vi "ReadREPL.vi"(8 "error in (no error)":errorcluster, 11 "Python":T1) -> (0 "error out":errorcluster, 1 "bytes read":u32, 2 "String":string, 3 "Python":T1)   [LabVIEW 2022 SP3]
uses:
  PythonCtrl.ctl
  Processors.ctl
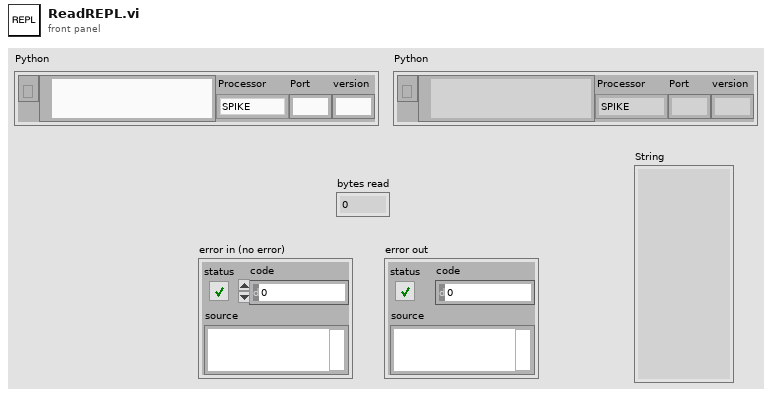
[diagram p1: front panel]
types:
  T1 = typedef "PythonCtrl.ctl" = cluster{"session":refnum<k35>, "PyPath":path, "Processor":T2, "Port":string, "version":string}
  T2 = typedef "Processors.ctl" = enum16{"SPIKE", "Pi", "Pi_ssh", "OpenMV", "Dunio"}
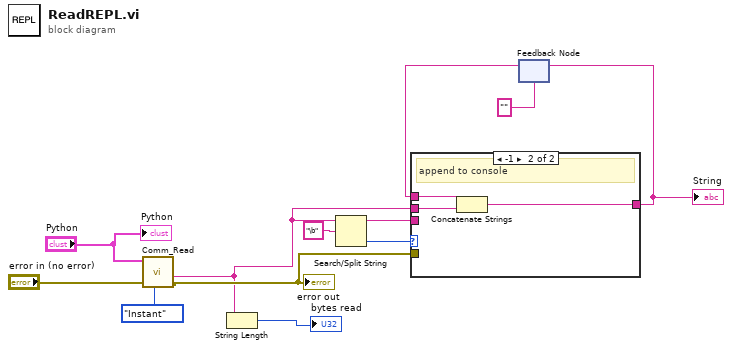
[diagram p0: block diagram]
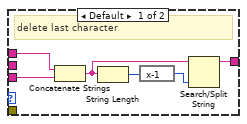
[diagram p2: hidden frame]
diagram:
  n1 = call "Comm_Read.vi"("Task"=enum16{"Instant", "All"}."Instant", "error in (no error)"="error in (no error)", "Python"="Python") -> ("error out"=w11:errorcluster, "Text read"=w6:string)  [unwired: 7 in]
  "error out" <- w11
  n2 = String Length(string=w6) -> (length=→"bytes read":i32)
  n3 = Search/Split String(string=w6, search string/char (-)="\b") -> (substring before match=w8:string, offset of match=w7:i32)  [unwired: 1 in, 1 out]
  n4 = feedback #1("") -> (w12:string)
  n5 = case shown="-1" w7 {
    tunnel: w8 -> [w13 _]
    tunnel: w6 -> [_ w19]
    tunnel: [w15 w21] -> w3
    tunnel: w11 -> [_ _]
    tunnel: w12 -> [w14 w20]
    frame Default {
      # "delete last character"
      n6 = Concatenate Strings(w14, w13) -> (w16:string)
      n7 = String Length(string=w16) -> (length=w17:i32)
      n8 = expression code="x-1"(w17) -> (w18:i32)
      n9 = Search/Split String(string=w16, offset (0)=w18) -> (substring before match=w15:string)  [unwired: 1 in, 2 out]
    }
    frame -1 {
      # "append to console"
      n10 = Concatenate Strings(w20, w19) -> (w21:string)
    }
  }
  "String" <- w3
  n11 = feedback-in #1(w3) -> ()
  "Python" <- "Python"
